vi "TDT-Get Target Val.vi"(0 "Data":T1={"TTankX"=refnum, "TDevAccX"=refnum, "LastTime"=0.0, "error"={"status"=FALSE, "code"=0, "source"=""}, "Block Name"="", "Circuit Tag"="", "Tank Name"="", "NumTicks"=0, "LastTick"=0.0, "Idle?"=FALSE, "Wait (ms)"=1000, "LastArtf"=0.0, "LastTosc"=0.0}, 7 "Target":string, 11 "error in (no error)":errorcluster) -> (8 "GetTargetVal":dbl, 15 "error out":errorcluster)   [LabVIEW 2015]
uses:
  TDT Interface Data.ctl
panel:
  in  "Default":dbl=nan
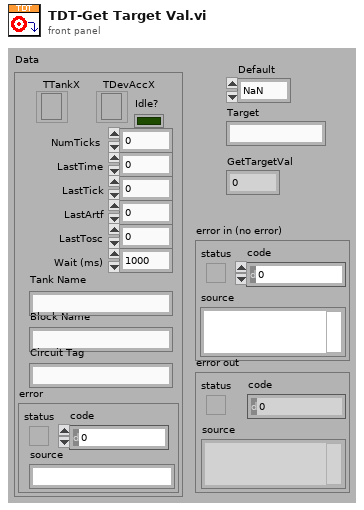
[diagram p1: front panel]
types:
  T1 = typedef "TDT Interface Data.ctl" = cluster{"TTankX":refnum<k7>, "TDevAccX":refnum<k7>, "LastTime":dbl, "error":errorcluster, "Block Name":string, "Circuit Tag":string, "Tank Name":string, "NumTicks":i32, "LastTick":dbl, "Idle?":bool, "Wait (ms)":u32, "LastArtf":dbl, "LastTosc":dbl}
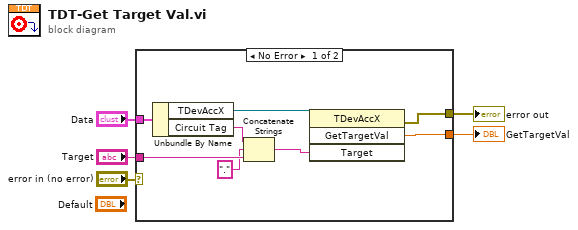
[diagram p0: block diagram]
diagram:
  n1 = case shown="No Error" "error in (no error)" {
    selector: "error in (no error)" -> [_ w14]
    tunnel: [w11 w14] -> w4
    tunnel: "Data" -> [w12 _]
    tunnel: "Target" -> [w9 _]
    tunnel: [w6 _] -> w1
    frame No Error {
      n2 = Unbundle By Name(w12) -> ("TDevAccX"=w13:refnum<k7>, "Circuit Tag"=w10:string)
      n3 = Concatenate Strings(w10, "." ("string"), w9) -> (w7:string)
      n4 = invoke class="TDevAccX" method="GetTargetVal"(reference=w13, "Target"=w7) -> (error out=w11:errorcluster, "GetTargetVal"=w6:dbl)  [unwired: 2 in, 2 out]
    }
    frame Error {
    }
  }
  "error out" <- w4
  "GetTargetVal" <- w1
